vi "WriteRealTimeStatus.vi"(8 "error in (no error)":errorcluster, 9 "DataGroups ChannelStatus in":T5[](array[typedef]), 10 "data in":T1) -> (0 "error out":errorcluster, 1 "DataGroups ChannelStatus out":T5[](array[typedef]), 2 "data out":T1)   [LabVIEW 2017, in "McsaTestPanel.lvlib"]
uses:
  <vilib>/addons/InsightCM/Devices/Shared/Mcsa/McsaTestPanel/McsaTestPanel.lvlib
  <vilib>/addons/InsightCM/Devices/Shared/Common/DataFlow/controls/Data.ctl
  <vilib>/addons/InsightCM/Utilities/DataAccessors/controls/wfmSGL_DVR.ctl
  <vilib>/addons/PointValueMap/controls/PointMap.ctl
  <vilib>/addons/InsightCM/Devices/Shared/Common/DataFlow/controls/Type.ctl
  <vilib>/addons/InsightCM/Devices/Shared/Mcsa/McsaTestPanel/controls/ChannelStatus.ctl
  <vilib>/addons/InsightCM/MessageBus/Base/controls/KeyValuePair.ctl
  <vilib>/addons/PointValueMap/PointValueMap.lvlib
  <vilib>/addons/InsightCM/Devices/Shared/Common/DataFlow/DataFlow.lvlib
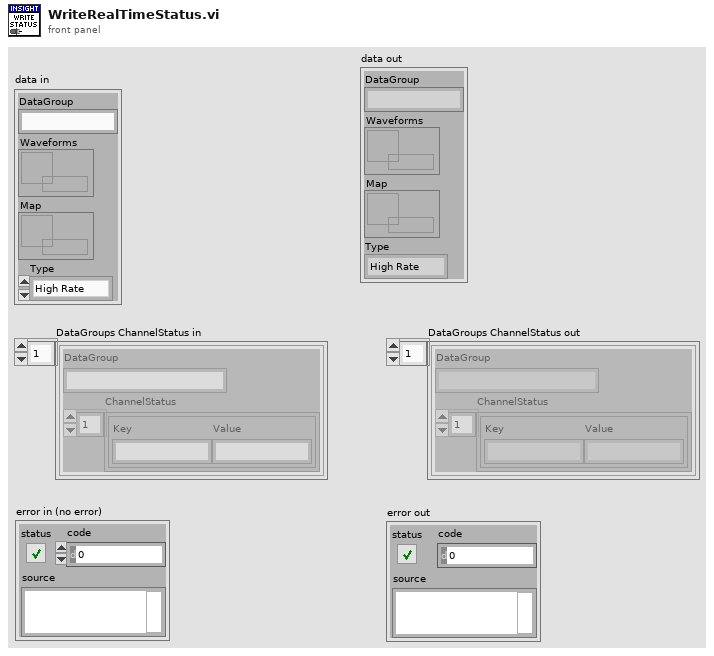
[diagram p1: front panel]
types:
  T1 = typedef "DataFlow.lvlib/Data.ctl" = cluster{"DataGroup":string, "Waveforms":T2, "Map":T3, "Type":T4}
  T2 = typedef "wfmSGL_DVR.ctl" = refnum<data-value>
  T3 = typedef "PointValueMap.lvlib/PointMap.ctl" = refnum<data-value>
  T4 = typedef "DataFlow.lvlib/Type.ctl" = enum16{"High Rate", "Low Rate", "Burst Mode"}
  T5 = typedef "McsaTestPanel.lvlib/ChannelStatus.ctl" = cluster{"DataGroup":string, "ChannelStatus":T6[]}
  T6 = typedef "KeyValuePair.ctl" = cluster{"Key":string, "Value":string}
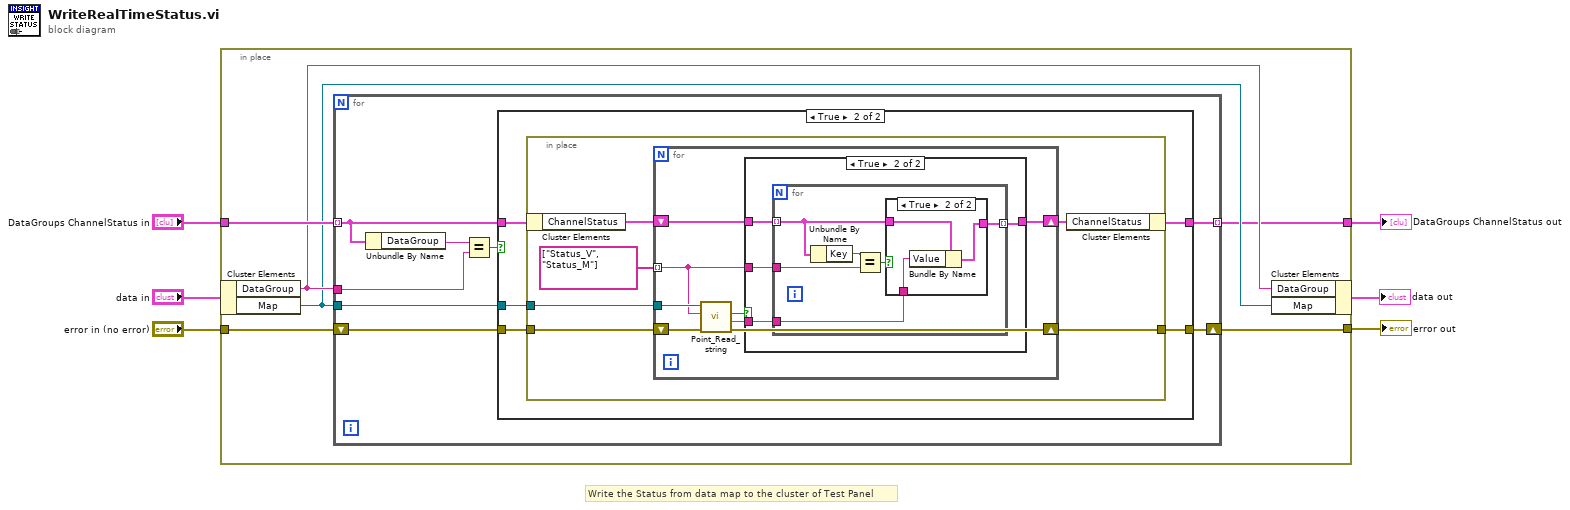
[diagram p0: block diagram]
diagram:
  # "Write the Status from data map to the cluster of Test Panel"
  n1 = in-place {
    in-place-border: "DataGroups ChannelStatus in" -> [w12]
    in-place-border: "error in (no error)" -> [w9]
    in-place-border: [w8] -> w3
    in-place-border: [w7] -> w2
    n2 = in-place-cluster #1("data in") -> ("DataGroup"=w11:string, "Map"=w10:T3)
    n3 = for {
      tunnel: w12 -> [w17] mode=indexing
      tunnel: w11 -> [w19]
      tunnel: w10 -> [w16]
      shift-right: [w14] -> w8
      shift-left: w9 -> [w15]
      tunnel: [w13] -> w7 mode=indexing
      n4 = Unbundle By Name(w17) -> ("DataGroup"=w20:string)
      n5 = Equal?(x=w20, y=w19) -> (x = y?=w18:bool)
      n6 = case shown="True" w18 {
        tunnel: w17 -> [w21 w27]
        tunnel: w16 -> [_ w26]
        tunnel: w15 -> [w22 w25]
        tunnel: [w22 w24] -> w14
        tunnel: [w21 w23] -> w13
        frame False {
        }
        frame True {
          n7 = in-place {
            in-place-border: w26 -> [w33]
            in-place-border: w25 -> [w32]
            in-place-border: [w31] -> w24
            n8 = in-place-cluster #2(w27) -> ("ChannelStatus"=w30:T6[])
            n9 = for {
              tunnel: w33 -> [w41]
              tunnel: string[] ["Status_V", "Status_M"] -> [w35] mode=indexing
              shift-right: [w39] -> w31
              shift-left: w32 -> [w40]
              shift-right: [w34] -> w28
              shift-left: w30 -> [w37]
              n10 = call <vilib>:"Point_Read_string.vi"("Error In"=w40, "Tag"=w35, "Map"=w41) -> ("Error Out"=w39:errorcluster, "Value"=w36:string, "Found?"=w38:bool)  [unwired: 3 in, 3 out]
              n11 = case shown="True" w38 {
                tunnel: w37 -> [w42 w46]
                tunnel: w36 -> [_ w43]
                tunnel: w35 -> [_ w45]
                tunnel: [w42 w44] -> w34
                frame False {
                }
                frame True {
                  n12 = for {
                    tunnel: w46 -> [w49] mode=indexing
                    tunnel: w45 -> [w51]
                    tunnel: [w50] -> w44 mode=indexing
                    tunnel: w43 -> [w47]
                    n13 = Unbundle By Name(w49) -> ("Key"=w52:string)
                    n14 = Equal?(x=w52, y=w51) -> (x = y?=w48:bool)
                    n15 = case shown="True" w48 {
                      tunnel: [w53 w56] -> w50
                      tunnel: w49 -> [w53 w55]
                      tunnel: w47 -> [_ w54]
                      frame False {
                      }
                      frame True {
                        n16 = Bundle By Name(cluster=w55, "Value"=w54) -> (w56:T6)
                      }
                    }
                  }
                }
              }
            }
            n17 = in-place-cluster #2("ChannelStatus"=w28) -> (w23:T5)
          }
        }
      }
    }
    n18 = in-place-cluster #1("DataGroup"=w11, "Map"=w10) -> (→"data out":T1)
  }
  "error out" <- w3
  "DataGroups ChannelStatus out" <- w2
